vi "Configure Trigger.vi"(8 "error in (no error)":errorcluster {"code" format="%.0x"}, 9 "trigger holdoff (60.0E-9 s)":dbl=6e-08 caption="Trigger Holdoff (60.0E-9 s)" format="%^.2e", 10 "Trigger Type (Edge)":i32(ring)=1 items=["Edge", "Glitch", "TV", "AC Line", "Pattern", "Duration", "IIC", "Sequence"], 11 "VISA Resource Name":refnum<visa-resource-name>) -> (0 "error out":errorcluster {"code" format="%.0x"}, 3 "VISA Resource Name Out":refnum<visa-resource-name>)   [LabVIEW 2011, in "Agilent 546XX Series.lvlib"]
doc: "This VI configures the common values of the trigger subsystem. These values are the trigger type and holdoff.\n\nWhen you call ag546xx Read Waveform, ag546xx Read Waveform Measurement, ag546xx Read Min Max Waveform, or ag546xx Initiate Acquisition, the oscilloscope waits for a trigger. You specify the type of trigger for which the oscilloscope waits with the Trigger Type control. \n\nIf the oscilloscope requires multiple waveform acquisitions to build a complete waveform, it waits for the length of time you specify with the Holdoff value to elapse since the previous trigger. The oscilloscope then waits for the next trigger. Once the oscilloscope acquires a complete waveform, it returns to the Idle state.\n\nNotes:\n\n(1) After you call this VI, you must call the trigger configuration VI that corresponds to the Trigger Type you select to completely specify the trigger. For example, if you set the Trigger Type to Edge Trigger, you use the ag546xx Configure Edge Trigger Source VI to completely specify the trigger."
uses:
  Agilent 546XX Series.lvlib
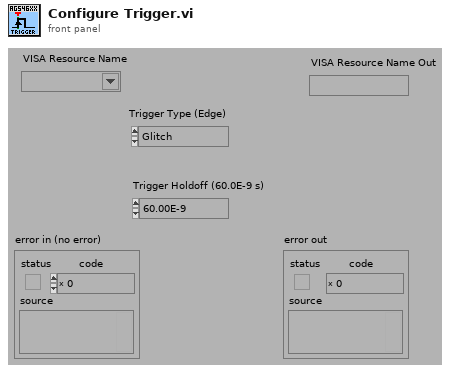
[diagram p1: front panel]
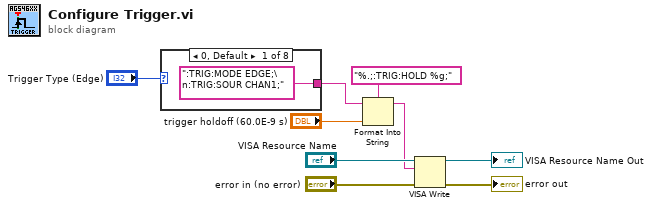
[diagram p0: block diagram]
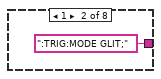
[diagram p2: hidden frame]
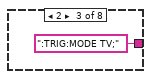
[diagram p3: hidden frame]
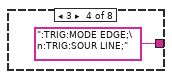
[diagram p4: hidden frame]
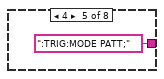
[diagram p5: hidden frame]
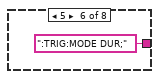
[diagram p6: hidden frame]
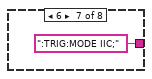
[diagram p7: hidden frame]
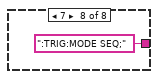
[diagram p8: hidden frame]
diagram:
  n1 = case shown="0, Default" "Trigger Type (Edge)" {
    tunnel: [":TRIG:MODE EDGE;\n:TRIG:SOUR CHAN1;" ":TRIG:MODE GLIT;" ":TRIG:MODE TV;" ":TRIG:MODE EDGE;\n:TRIG:SOUR LINE;" ":TRIG:MODE PATT;" ":TRIG:MODE DUR;" ":TRIG:MODE IIC;" ":TRIG:MODE SEQ;"] -> w2
    frame 0, Default {
    }
    frame 1 {
    }
    frame 2 {
    }
    frame 3 {
    }
    frame 4 {
    }
    frame 5 {
    }
    frame 6 {
    }
    frame 7 {
    }
  }
  n2 = Format Into String(format string="%.;:TRIG:HOLD %g;", initial string=w2, "trigger holdoff (60.0E-9 s)") -> (resulting string=w1:string)  [unwired: 1 in, 1 out]
  n3 = VISA Write(VISA resource name="VISA Resource Name", write buffer=w1, error in (no error)="error in (no error)") -> (VISA resource name out=→"VISA Resource Name Out":refnum<visa-resource-name>, error out=→"error out":errorcluster)  [unwired: 1 out]
